vi "ErrorDefinitionSQLite_Create.vi"(8 "ErrorIn":errorcluster caption="Error In(no Error)", 11 "Reference in":refnum<class "ErrorDefinitionSQLite.lvclass"> caption="Reference In") -> (0 "ErrorOut":errorcluster caption="Error Out", 3 "Reference out":refnum<class "ErrorDefinitionSQLite.lvclass"> caption="Reference Out")   [LabVIEW 2018, in "ErrorDefinitionSQLite.lvclass"]
uses:
  <userlib>/_express/CustomErrorCreator/ErrorDefinitionSQLite/ErrorDefinitionSQLite.lvclass
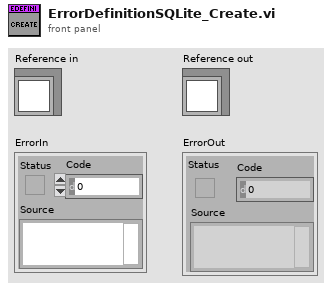
[diagram p1: front panel]
types:
  T1 = typedef "ErrorDefinitionSQLite.lvclass/ObjectAttributes.ctl" = cluster{"Path":path}
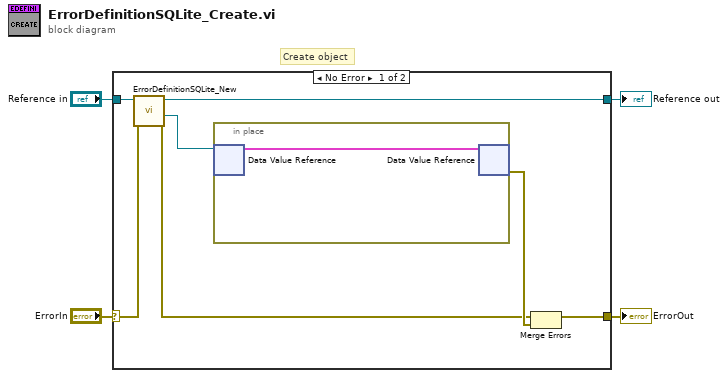
[diagram p0: block diagram]
diagram:
  # "Create object"
  n1 = case shown="No Error" "ErrorIn" {
    selector: "ErrorIn" -> [w10 w14]
    tunnel: [w6 w14] -> w3
    tunnel: "Reference in" -> [w11 w13]
    tunnel: [w9 w13] -> w1
    frame No Error {
      n2 = call <userlib>:"ErrorDefinitionSQLite_New.vi"("ErrorIn"=w10, "Reference in"=w11) -> ("ErrorOut"=w5:errorcluster, "DVRRefOut"=w7:refnum<data-value>, "Reference out"=w9:refnum<class "ErrorDefinitionSQLite.lvclass">)  [unwired: 6 in, 1 out]
      n3 = in-place "In Place Element Structure" {
        n4 = in-place-dvr #1(w7) -> (w12:T1)  [unwired: 1 out]
        n5 = in-place-dvr #1(w12) -> (w8:errorcluster)  [unwired: 1 out]
      }
      n6 = Merge Errors(w5, w8) -> (w6:errorcluster)
    }
    frame Error {
    }
  }
  "ErrorOut" <- w3
  "Reference out" <- w1
